vi "EventPassState.vi"(9 "TestPasse":bool[](array[boolean]), 10 "IA State Input":T1) -> (1 "Id":dbl, 2 "IA State Output":T1, 3 "Pass State":bool)   [LabVIEW 2017]
uses:
  Core/AI Input.ctl
  Core/AI Robot.ctl
  Intel/Functions Enum.ctl
  Intel/AttackerStates.ctl
  Path Planning/RRT/PathDests.ctl
  Path Planning/RRT/PathDest.ctl
  Core/AI Ball.ctl
  Core/Field Size.ctl
  Core/AI Judge.ctl
  Intel/Command Enum.ctl
  Events.ctl
panel:
  in  "Desabilita passe":bool=TRUE
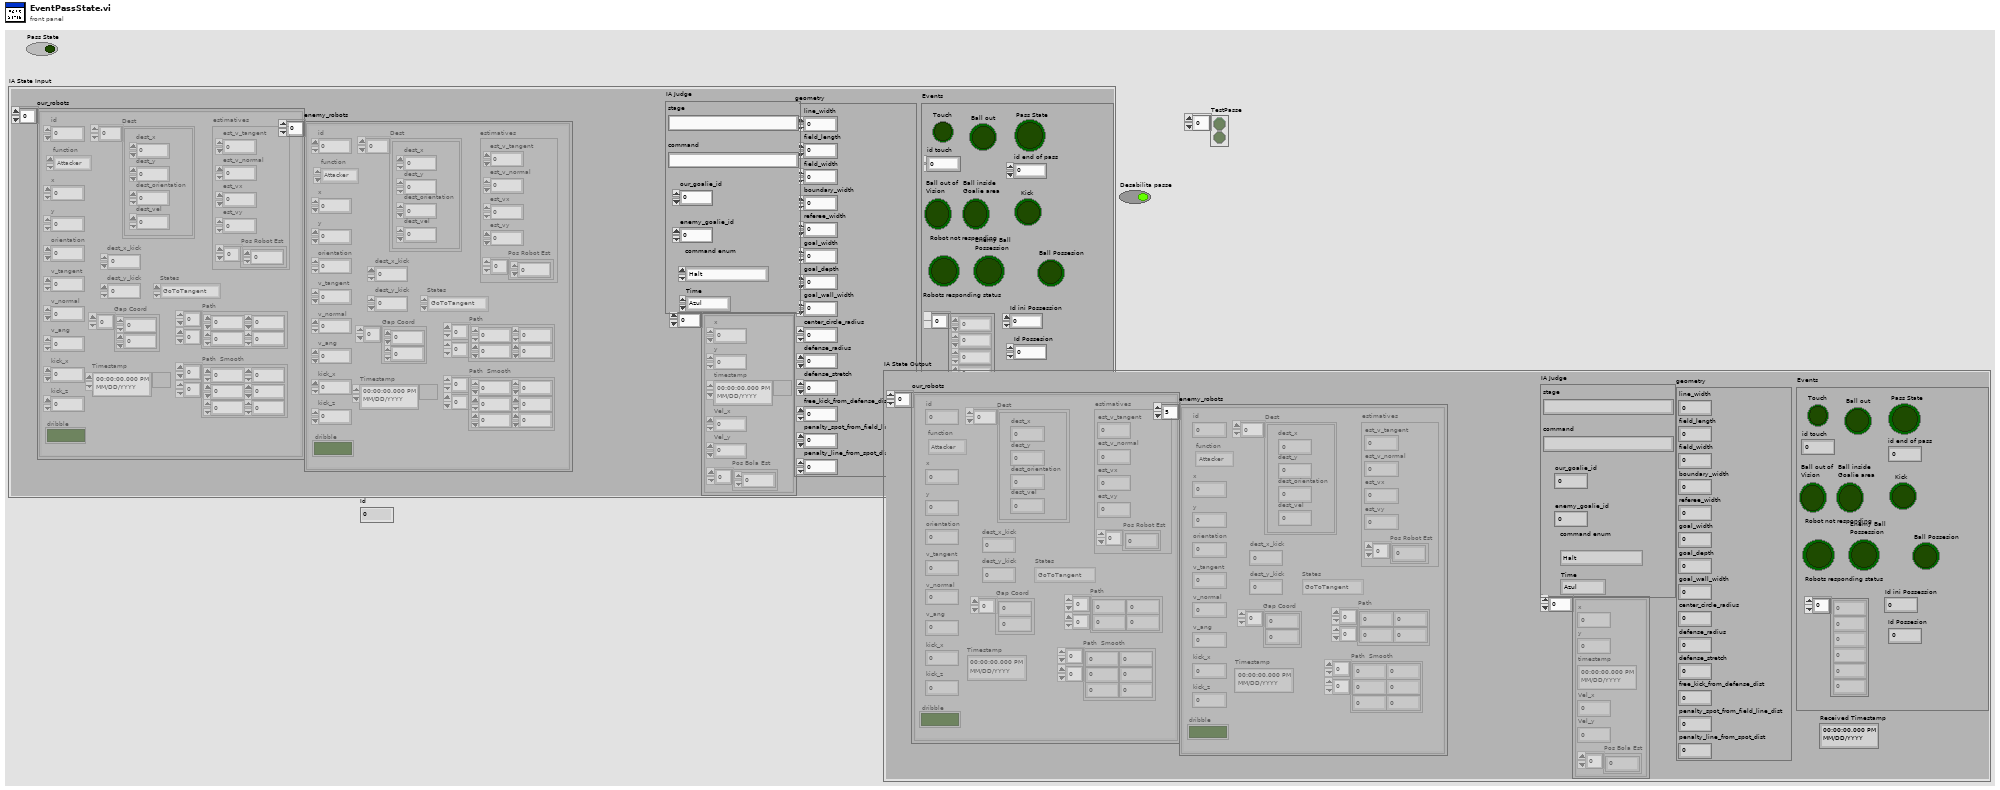
[diagram p1: front panel]
types:
  T1 = typedef "AI Input.ctl" = cluster{"our_robots":T2[], "enemy_robots":T2[], "balls":T7[], "geometry":T8, "IA Judge":T9, "Received Timestamp":timestamp, "Events":T11}
  T2 = typedef "AI Robot.ctl" = cluster{"id":u32, "function":T3, "x":dbl, "y":dbl, "orientation":dbl, "v_tangent":dbl, "v_normal":dbl, "v_ang":dbl, "kick_x":dbl, "kick_z":dbl, "dribble":bool, "Timestamp":timestamp, "estimatives":cluster{"est_v_tangent":dbl, "est_v_normal":dbl, "est_vx":dbl, "est_vy":dbl, "Pos Robot Est":dbl[]}, "dest_x_kick":dbl, "dest_y_kick":dbl, "Gap Coord":dbl[], "States":T4, "Path ":dbl[][], "Path  Smooth":dbl[][], "Dest":T5}
  T3 = typedef "Functions Enum.ctl" = enum16{"Attacker", "Goalie", "Defender", "Striker", "Goto 0", "Dummy", "Kicker", "ZigZag"}
  T4 = typedef "AttackerStates.ctl" = enum16{"Pass", "GoToTangent", "BallGetting", "GoToKick", ""}
  T5 = typedef "PathDests.ctl" = T6[]
  T6 = typedef "PathDest.ctl" = cluster{"dest_x":dbl, "dest_y":dbl, "dest_orientation":dbl, "dest_vel":dbl}
  T7 = typedef "AI Ball.ctl" = cluster{"x":dbl, "y":dbl, "timestamp":timestamp, "Vel_x":dbl, "Vel_y":dbl, "Pos Bola Est":dbl[]}
  T8 = typedef "Field Size.ctl" = cluster{"line_width":u32, "field_length":u32, "field_width":u32, "boundary_width":u32, "referee_width":u32, "goal_width":u32, "goal_depth":u32, "goal_wall_width":u32, "center_circle_radius":u32, "defense_radius":u32, "defense_stretch":u32, "free_kick_from_defense_dist":u32, "penalty_spot_from_field_line_dist":u32, "penalty_line_from_spot_dist":u32}
  T9 = typedef "AI Judge.ctl" = cluster{"stage":string, "command":string, "our_goalie_id":dbl, "enemy_goalie_id":dbl, "command enum":T10, "Time":enum16{"Azul", "Amarelo"}}
  T10 = typedef "Command Enum.ctl" = enum16{"Halt", "Stop", "Force Start", "PKA Normal Start", "Prepare Kickoff Ally", "PKE Normal Start", "Prepare Kickoff Enemy", "Prepare Penalty Ally", "PPA Normal Start", "Prepare Penalty Enemy", "PPE Normal Start", "Direct Free Enemy", "Direct Free Ally", "Indirect Free Enemy", "Indirect Free Ally", "Timeout Enemy", "Timeout Ally", "Goal Enemy", "Goal Ally", "Ball Placement Enemy", "Ball Placement Ally", "Normal Half Time", "Extra Time Break", "Extra Half Time", "None", "Post Game"}
  T11 = typedef "Events.ctl" = cluster{"Touch":bool, "Ball out":bool, "id touch":dbl, "Ball out of \nVision":bool, "Ball inside \nGoalie area":bool, "Robot not responding":bool, "Robots responding status":dbl[], "Enemy Ball \nPossession":bool, "Pass State":bool, "id end of pass":dbl, "Kick":bool, "Id ini Possession":dbl, "Ball Possesion":bool, "Id Possesion":dbl}
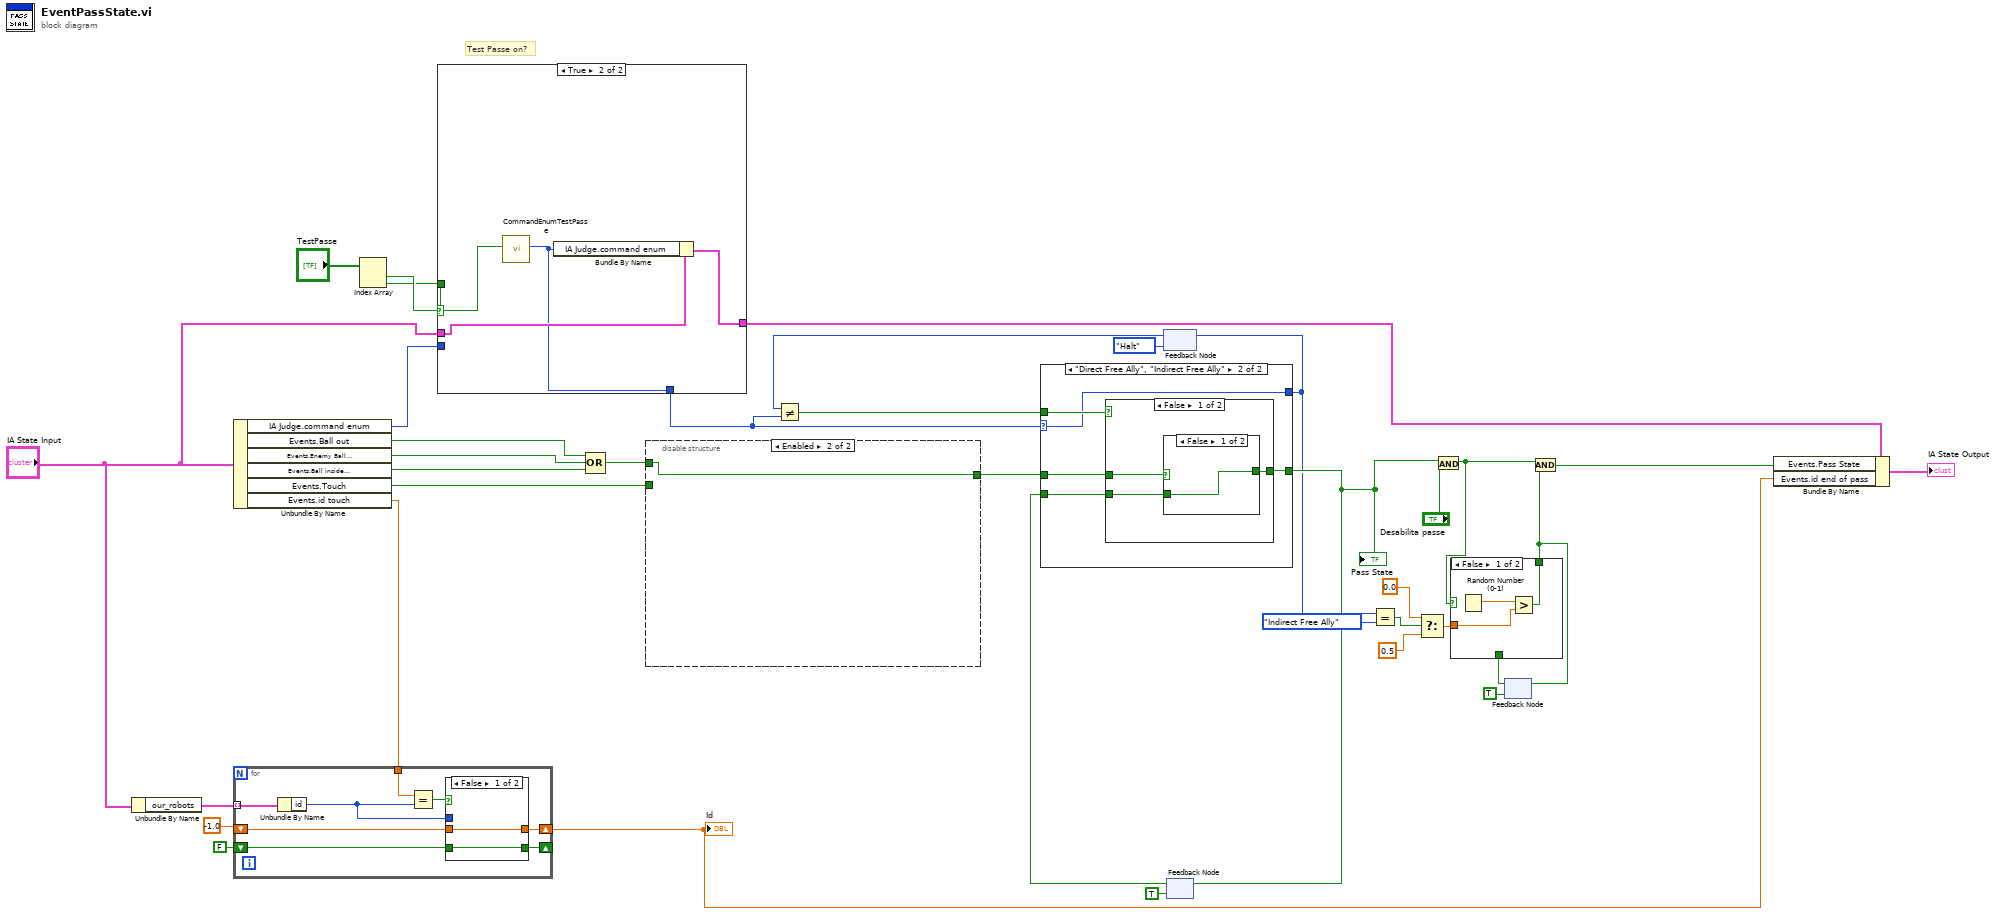
[diagram p0: block diagram]
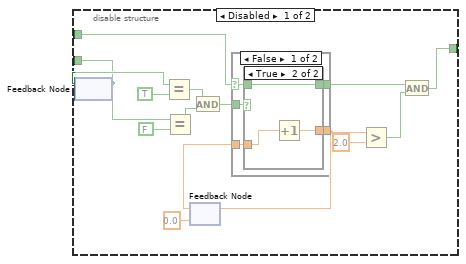
[diagram p4: hidden frame]
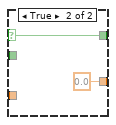
[diagram p6: hidden frame]
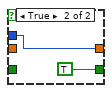
[diagram p7: hidden frame]
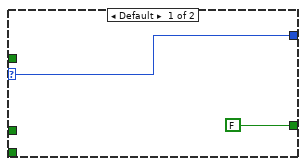
[diagram p8: hidden frame]
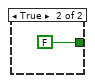
[diagram p9: hidden frame]
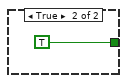
[diagram p10: hidden frame]
diagram:
  # "Test Passe on?"
  n1 = Unbundle By Name("IA State Input") -> ("our_robots"=w32:T2[])
  n2 = Unbundle By Name("IA State Input") -> ("IA Judge.command enum"=w5:T10, "Events.Ball out"=w25:bool, "Events.Enemy Ball \nPossession"=w24:bool, "Events.Ball inside \nGoalie area"=w23:bool, "Events.Touch"=w26:bool, "Events.id touch"=w31:dbl)
  n3 = for {
    tunnel: w32 -> [w45] mode=indexing
    shift-right: [w42] -> _
    shift-left: FALSE -> [w43]
    tunnel: w31 -> [w44]
    shift-right: [w39] -> w27
    shift-left: -1.0 -> [w38]
    n4 = Unbundle By Name(w45) -> ("id"=w40:u32)
    n5 = Equal?(x=w44, y=w40) -> (x = y?=w41:bool)
    n6 = case shown="False" w41 {
      tunnel: w43 -> [w47 _]
      tunnel: [w47 TRUE] -> w42
      tunnel: w40 -> [_ w48]
      tunnel: [w46 w48] -> w39
      tunnel: w38 -> [w46 _]
      frame False {
      }
      frame True {
      }
    }
  }
  "Id" <- w27
  n7 = Index Array(array="TestPasse") -> (element #1=w6:bool, element #2=w3:bool)  [unwired: 2 in]
  n8 = case shown="True" w6 {
    tunnel: w5 -> [w51 _]
    tunnel: [w51 w52] -> w4
    tunnel: w3 -> [_ w55]
    tunnel: "IA State Input" -> [w50 w54]
    tunnel: [w50 w53] -> w1
    frame False {
    }
    frame True {
      n9 = call "CommandEnumTestPasse.vi"("Reset"=w55) -> ("command enum"=w52:T10)  [unwired: 10 in]
      n10 = Bundle By Name(cluster=w54, "IA Judge.command enum"=w52) -> (w53:T1)
    }
  }
  n11 = Compound Arithmetic op=OR(w25, w24, w23) -> (w22:bool)
  n12 = disable-structure shown="Enabled" {
    disable-tunnel: w26 -> [w69 _]
    disable-tunnel: w22 -> [w59 w83]
    disable-tunnel: [w56 w83] -> w21
    frame Disabled {
      n13 = feedback #1() -> (w70:bool)  [unwired: 1 in]
      n14 = feedback-in #1(w69) -> ()
      n15 = Equal?(x=w70, y=TRUE) -> (x = y?=w66:bool)
      n16 = Equal?(x=w69, y=FALSE) -> (x = y?=w65:bool)
      n17 = feedback #2(0.0) -> (w63:dbl)
      n18 = And(x=w66, y=w65) -> (x .and. y?=w64:bool)
      n19 = case shown="False" w59 {
        selector: w59 -> [w72 w81]
        tunnel: w64 -> [w75 _]
        tunnel: w63 -> [w74 _]
        tunnel: [w73 0.0] -> w61
        tunnel: [w71 w81] -> w57
        frame False {
          n20 = case shown="True" w75 {
            tunnel: [w77 w80] -> w73
            tunnel: w74 -> [w77 w79]
            tunnel: w72 -> [w76 w78]
            tunnel: [w76 w78] -> w71
            frame False {
            }
            frame True {
              n21 = Increment(x=w79) -> (x+1=w80:dbl)
            }
          }
        }
        frame True {
        }
      }
      n22 = feedback-in #2(w61) -> ()
      n23 = Greater?(x=w61, y=2.0) -> (0:w58:bool)
      n24 = And(x=w57, y=w58) -> (x .and. y?=w56:bool)
    }
    frame Enabled {
    }
  }
  n25 = feedback #3(Command_Enum."Halt" ("command\nenum")) -> (w37:T10)
  n26 = Not Equal?(x=w37, y=w4) -> (x != y?=w36:bool)
  n27 = feedback #4(TRUE) -> (w35:bool)
  n28 = case shown="\"Direct Free Ally\", \"Indirect Free Ally\"" w4 {
    selector: w4 -> [w84 w86]
    tunnel: w21 -> [_ w90]
    tunnel: w36 -> [_ w89]
    tunnel: [FALSE w88] -> w20
    tunnel: w35 -> [_ w87]
    tunnel: [w84 w86] -> w13
    frame Default {
    }
    frame "Direct Free Ally", "Indirect Free Ally" {
      n29 = case shown="False" w89 {
        tunnel: w90 -> [w93 _]
        tunnel: [w92 TRUE] -> w88
        tunnel: w87 -> [w91 _]
        frame False {
          n30 = case shown="False" w93 {
            tunnel: [w94 FALSE] -> w92
            tunnel: w91 -> [w94 _]
            frame False {
            }
            frame True {
            }
          }
        }
        frame True {
        }
      }
    }
  }
  "Pass State" <- w20
  n31 = feedback-in #3(w13) -> ()
  n32 = feedback-in #4(w20) -> ()
  n33 = Equal?(x=w13, y=Command_Enum."Indirect Free Ally") -> (x = y?=w10:bool)
  n34 = Select(t=0.0, s=w10, f=0.5 ("y")) -> (s? t:f=w8:dbl)
  n35 = And(x=w20, y="Desabilita passe") -> (x .and. y?=w17:bool)
  n36 = feedback #5(TRUE) -> (w16:bool)
  n37 = case shown="False" w17 {
    tunnel: [w98 w100] -> w14
    tunnel: w16 -> [_ w100]
    tunnel: w8 -> [w97 _]
    frame False {
      n38 = Random Number (0-1)() -> (number: 0 to 1=w99:dbl)
      n39 = Greater?(x=w99, y=w97) -> (0:w98:bool)
    }
    frame True {
    }
  }
  n40 = feedback-in #5(w14) -> ()
  n41 = And(x=w17, y=w14) -> (x .and. y?=w18:bool)
  n42 = Bundle By Name(cluster=w1, "Events.Pass State"=w18, "Events.id end of pass"=w27) -> (→"IA State Output":T1)
